vi "Reset Child Text.vi"(8 "Tag":string, 10 "Multi-Item Text":cluster{"Array":string[]}[](array[cluster]), 11 "Tree in":refnum<class "Tree.lvclass">) -> (3 "Tree out":refnum<class "Tree.lvclass">)   [LabVIEW 2024, in "Tree.lvclass"]
uses:
  Tree.lvclass
  Tree.lvclass/Tree.ctl
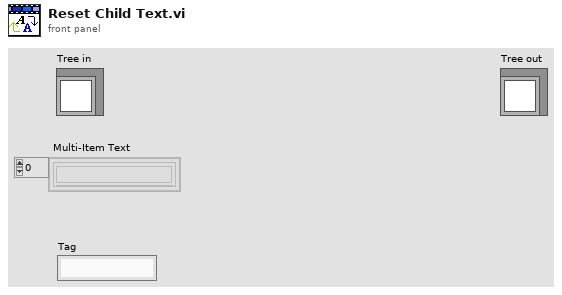
[diagram p1: front panel]
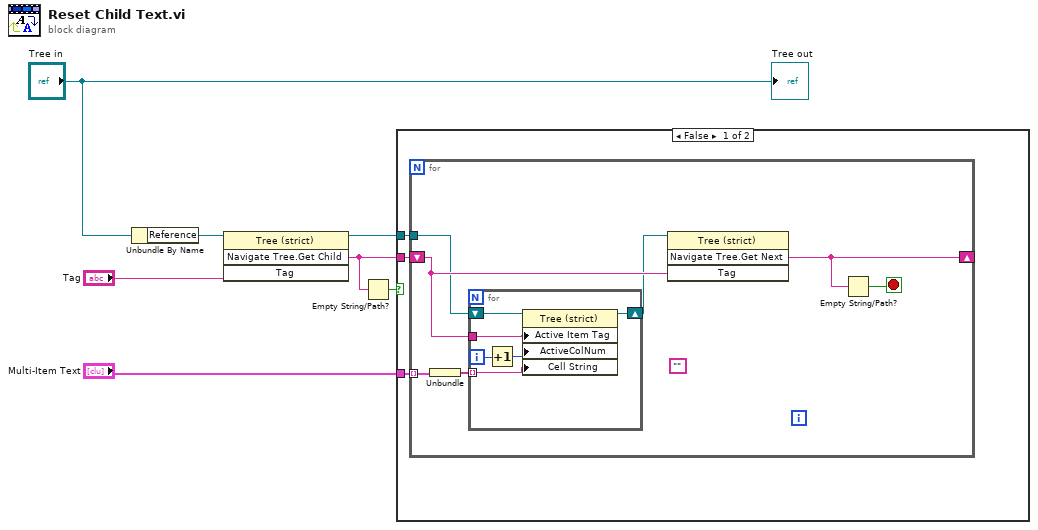
[diagram p0: block diagram]
diagram:
  n1 = Unbundle By Name("Tree in") -> ("Reference"=w7:refnum<vi>)
  n2 = invoke class="Tree (strict)" method="Navigate Tree.Get Child"(reference=w7, "Tag"="Tag") -> (reference out=w5:refnum<vi>, "Navigate Tree:Get Child"=w2:string)  [unwired: 2 in, 2 out]
  n3 = Empty String/Path?(string/path=w2) -> (empty?=w1:bool)
  n4 = case shown="False" w1 {
    tunnel: w5 -> [w10 _]
    tunnel: "Multi-Item Text" -> [w9 _]
    tunnel: w2 -> [w8 _]
    frame False {
      n5 = for {
        shift-right: [w14] -> _
        shift-left: w8 -> [w17]
        tunnel: w10 -> [w15]
        tunnel: w9 -> [w12] mode=indexing
        stop <- w13 stop-if-true
        (unwired) ""
        n6 = Unbundle(w12) -> ("Array"=w11:string[])
        n7 = for {
          tunnel: w17 -> [w23]
          shift-right: [w22] -> w16
          shift-left: w15 -> [w21]
          tunnel: w11 -> [w18] mode=indexing
          i -> [w19]
          n8 = Increment(x=w19) -> (x+1=w20:i32)
          n9 = property class="Tree (strict)"(reference=w21, "Active Item Tag"=w23, "ActiveColNum"=w20, "Cell String"=w18) -> (reference out=w22:refnum<vi>)  [unwired: 1 in, 1 out]
        }
        n10 = invoke class="Tree (strict)" method="Navigate Tree.Get Next"(reference=w16, "Tag"=w17) -> ("Navigate Tree:Get Next Item"=w14:string)  [unwired: 2 in, 3 out]
        n11 = Empty String/Path?(string/path=w14) -> (empty?=w13:bool)
      }
    }
    frame True {
    }
  }
  "Tree out" <- "Tree in"
